vi "RT Main_Write Bool Cluster.vi"() -> ()   [LabVIEW 2018]
uses:
  Speciality IO/Types/Static.Generate.Digital.Settings.ctl
  Speciality IO/Types/Static.Measure.Digital.Measurement.ctl
  58ef3a2b-dcb5-4c85-9d81-a61eb9170448.vi
  c2afd2a8-09c3-412a-8e32-3b07695bb373.vi
  FPGA Bitfile Register Operations/Scalar IO Operations/SubVIs/Parse Cluster Configuration.vi
  FPGA Bitfile Register Operations/Scalar IO Operations/Write Methods/Write Data Register/Instances/Write U8 Array.vi
  FPGA Bitfile Register Operations/Scalar IO Operations/Read Methods/Read Data Register/Instances/Read U8 Array.vi
  FPGA Bitfile Register Operations/Scalar IO Operations/SubVIs/Check Cluster Configuration Store.vi
  FPGA Bitfile Register Operations/Scalar IO Operations/Utilities/Find Register Offset.vi
  FPGA Bitfile Register Operations/Scalar IO Operations/SubVIs/Check Register Data Store.vi
  <userlib>/_OpenG.lib/lvdata/lvdata.llb/Variant to Header Info__ogtk.vi
  <userlib>/_OpenG.lib/lvdata/lvdata.llb/Split Cluster TD__ogtk.vi
  <userlib>/_OpenG.lib/lvdata/lvdata.llb/Cluster to Array of VData__ogtk.vi
  <vilib>/Utility/Data Type/Get Type Information.vi
  <userlib>/_OpenG.lib/lvdata/lvdata.llb/Get Strings from Enum__ogtk.vi
  FPGA Bitfile Register Operations/Scalar IO Operations/Error Handling/Error 6004.vi
  <vilib>/Utility/Data Type/Get Fixed-Point Information.vi
  FPGA Bitfile Register Operations/Scalar IO Operations/Error Handling/Error 6001.vi
  FPGA Bitfile Register Operations/Scalar IO Operations/Error Handling/Error 6000.vi
  FPGA Bitfile Register Operations/Scalar IO Operations/Error Handling/Error 6002.vi
  FPGA Bitfile Register Operations/Scalar IO Operations/Error Handling/Error 6006.vi
  FPGA Bitfile Register Operations/Scalar IO Operations/Error Handling/Error 6003.vi
  <vilib>/FPGAPlugInAG/Dynamic/niLvFpga_Close_Dynamic.vi
  <vilib>/rvi/interface/nirviCloseFPGA/nirviCloseFPGA.xnode
  FPGA Bitfile Register Operations/Scalar IO Operations/FPGA Register IO.lvlib
  Speciality IO/Speciality FPGA IO.lvlib
panel:
  out "Measurement (read)":T1
  in  "Settings (write)":T2={"ACTIVE EDGE"=TRUE, "OUTPUT"=FALSE}
  out "Average seconds per read":dbl
  out "error out":errorcluster
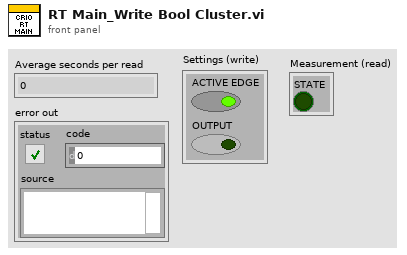
[diagram p1: front panel]
types:
  T1 = typedef "Speciality FPGA IO.lvlib/Static.Measure.Digital.Measurement.ctl" = cluster{"STATE":bool}
  T2 = typedef "Speciality FPGA IO.lvlib/Static.Generate.Digital.Settings.ctl" = cluster{"ACTIVE EDGE":bool, "OUTPUT":bool}
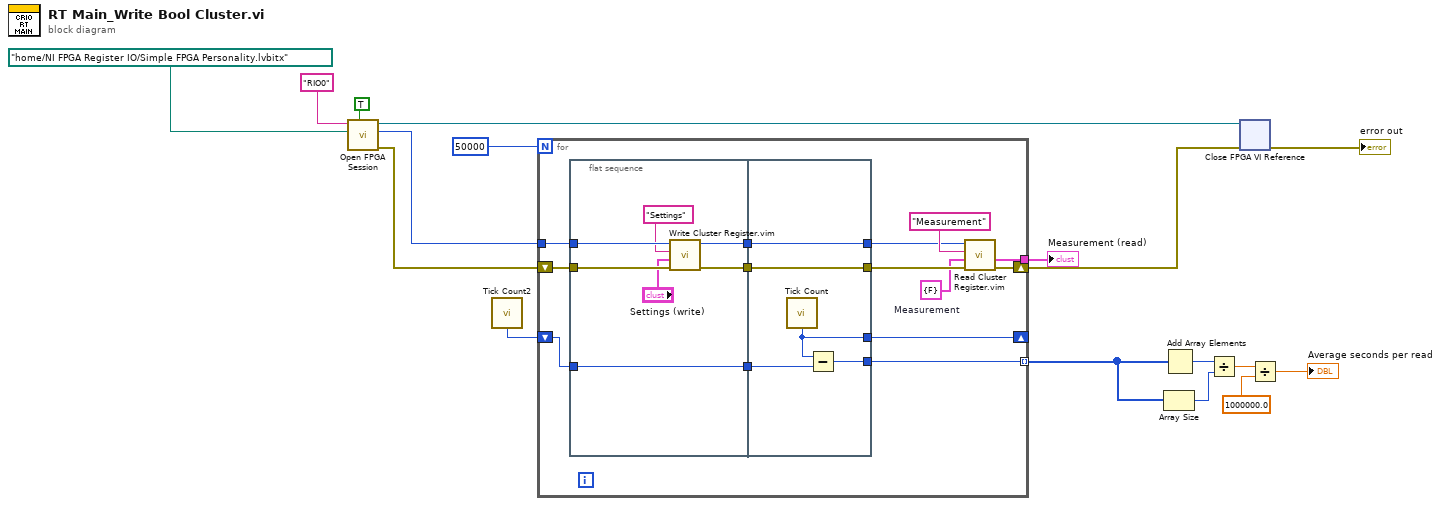
[diagram p0: block diagram]
diagram:
  n1 = call "Open FPGA Session.vi"("run when loaded (T)"=TRUE ("Run When Loaded (T)"), "bitfile path"=path "/home/NI FPGA Register IO/Simple FPGA Personality.lvbitx" ("Bitfile path"), "device address"="RIO0" ("Device address")) -> ("error out"=w4:errorcluster, "session out"=w3:u32, "bitfile reference out"=w14:refnum<k20>)  [unwired: 6 in]
  n2 = call "Tick Count2"() -> ("Tick Count(uSec)"=w11:u32)
  n3 = for {
    N: 50000 -> [_]
    shift-right: [w22] -> w2
    shift-left: w4 -> [w31]
    shift-right: [w28] -> _
    shift-left: w11 -> [w30]
    tunnel: [w27] -> w10 mode=indexing
    tunnel: w3 -> [w26]
    tunnel: [w18] -> w1
    w19 = T1 {"STATE"=FALSE}  # Measurement
    n4 = flat-sequence {
      tunnel: w31 -> [w36]
      tunnel: w30 -> [w38]
      tunnel: [w38] -> w29
      tunnel: w26 -> [w37]
      tunnel: [w34] -> w25
      tunnel: [w33] -> w21
      tunnel: w29 -> [w43]
      tunnel: w25 -> [w40]
      tunnel: [w42] -> w28
      tunnel: [w41] -> w27
      tunnel: [w40] -> w23
      tunnel: w21 -> [w39]
      tunnel: [w39] -> w20
      frame #0 {
        n5 = call "Write Cluster Register.vim"("error in (no error)"=w36, "Cluster in"="Settings (write)", "Cluster Name"="Settings" ("register name"), "session in"=w37) -> ("error out"=w34:errorcluster, "session out"=w33:u32)  [unwired: 6 in]
      }
      frame #1 {
        n6 = call "Tick Count"() -> ("Tick Count(uSec)"=w42:u32)
        n7 = Subtract(x=w42, y=w43) -> (x-y=w41:u32)
      }
    }
    n8 = call "Read Cluster Register.vim"("error in (no error)"=w23, "Cluster in (default value)"=w19, "Cluster Name"="Measurement", "session in"=w20) -> ("error out"=w22:errorcluster, "Cluster out"=w18:T1)  [unwired: 5 in, 1 out]
  }
  "Measurement (read)" <- w1
  n9 = Array Size(array=w10) -> (size(s)=w8:i32)
  n10 = Add Array Elements(numeric array=w10) -> (sum=w9:u32)
  n11 = Divide(x=w9, y=w8) -> (x/y=w7:dbl)
  n12 = xnode "Close FPGA VI Reference"("FPGA VI Reference In"=w14, "error in"=w2) -> ("error out"=→"error out":errorcluster)
  n13 = Divide(x=w7, y=1000000.0) -> (x/y=→"Average seconds per read":dbl)
